vi "CompareVersions.vi"(0 "robotPolyScopeVersion":T1, 5 "commandMinVersion":T1) -> (14 "compatible":bool)   [LabVIEW 2016, in "Universal Robot.lvclass"]
uses:
  Universal Robot.lvclass
  PolyScopeVersion.ctl
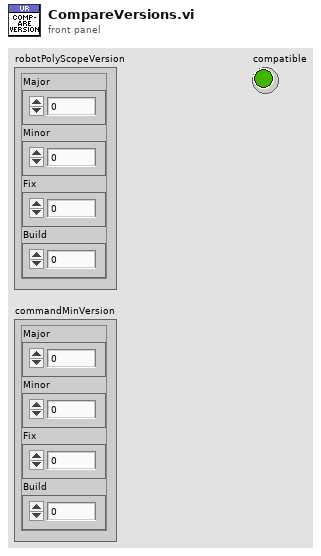
[diagram p1: front panel]
types:
  T1 = typedef "Universal Robot.lvclass/PolyScopeVersion.ctl" = cluster{"Major":i32, "Minor":i32, "Fix":i32, "Build":i32}
  T2 = cluster{"Major":bool, "Minor":bool, "Fix":bool, "Build":bool}
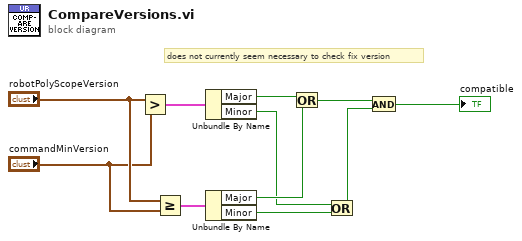
[diagram p0: block diagram]
diagram:
  # "does not currently seem necessary to check fix version"
  n1 = Greater?(x="robotPolyScopeVersion", y="commandMinVersion") -> (0:w11:T2)
  n2 = Greater Or Equal?(x="robotPolyScopeVersion", y="commandMinVersion") -> (x >= y?=w8:T2)
  n3 = Unbundle By Name(w11) -> ("Major"=w7:bool, "Minor"=w5:bool)
  n4 = Unbundle By Name(w8) -> ("Major"=w6:bool, "Minor"=w4:bool)
  n5 = Or(x=w7, y=w6) -> (x .or. y?=w3:bool)
  n6 = Or(x=w5, y=w4) -> (x .or. y?=w2:bool)
  n7 = And(x=w3, y=w2) -> (x .and. y?=→"compatible":bool)
